vi "Measurement.SetConfiguration.vi"(8 "error in (no error)":errorcluster, 10 "Configuration":variant, 11 "Measurement.WavelengthSweeping in":refnum<class "Measurement.WavelengthSweeping.lvclass">) -> (0 "error out":errorcluster, 3 "Measurement.WavelengthSweeping out":refnum<class "Measurement.WavelengthSweeping.lvclass">)   [LabVIEW 2017, in "Measurement.WavelengthSweeping.lvclass"]
uses:
  Measurement.WavelengthSweeping.lvclass
  Typedefs/Configuration--Cluster.ctl
  Measurement/Typedefs/Measurement.Type--Enum.ctl
  Typedefs/Configuration.Hardware--Cluster.ctl
  Measurement/Typedefs/Configuration.SMU--Cluster.ctl
  SMU/Typedefs/Configuration--Cluster.ctl
  Measurement/Typedefs/Configuration.LIA--Cluster.ctl
  LIA/Typedefs/Configuration--Cluster.ctl
  Measurement/Typedefs/Configuration.OPM--Cluster.ctl
  OPM/Typedefs/Configuration--Cluster.ctl
  Measurement/Typedefs/Configuration.OPA--Cluster.ctl
  OPA/Typedefs/Configuration--Cluster.ctl
  Typedefs/Configuration.Measurement--Cluster.ctl
  Measurement/Measurement.lvclass
  SMU/SMU.lvclass
  LIA/LIA.lvclass
  OPM/OPM.lvclass
  OPA/OPA.lvclass
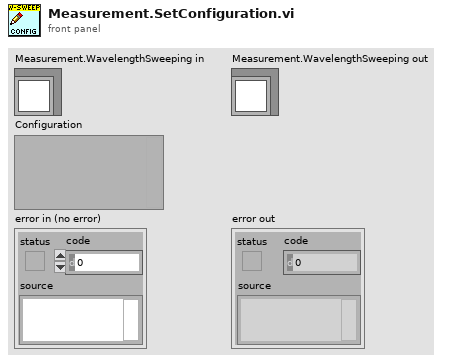
[diagram p1: front panel]
types:
  T1 = typedef "Measurement.WavelengthSweeping.lvclass/Configuration--Cluster.ctl" = cluster{"Measurement.Type":T2, "Hardware":T3, "Measurement":T12}
  T2 = typedef "Measurement.lvclass/Measurement.Type--Enum.ctl" = enum16{"Free", "I/V Curve", "Wavelength sweeping", "Photocurrent mapping"}
  T3 = typedef "Measurement.WavelengthSweeping.lvclass/Configuration.Hardware--Cluster.ctl" = cluster{"SMU":T4, "LIA":T6, "OPM":T8, "OPA":T10}
  T4 = typedef "Measurement.lvclass/Configuration.SMU--Cluster.ctl" = cluster{"Enable":bool, "SMU Model":string, "Configuration":T5}
  T5 = typedef "SMU.lvclass/Configuration--Cluster.ctl" = cluster{"VISA Resource":string, "Channel":string}
  T6 = typedef "Measurement.lvclass/Configuration.LIA--Cluster.ctl" = cluster{"Enable":bool, "LIA Model":string, "Configuration":T7}
  T7 = typedef "LIA.lvclass/Configuration--Cluster.ctl" = cluster{"VISA Resource":string}
  T8 = typedef "Measurement.lvclass/Configuration.OPM--Cluster.ctl" = cluster{"Enable":bool, "OPM Model":string, "Configuration":T9}
  T9 = typedef "OPM.lvclass/Configuration--Cluster.ctl" = cluster{"VISA Resource":string}
  T10 = typedef "Measurement.lvclass/Configuration.OPA--Cluster.ctl" = cluster{"Enable":bool, "OPA Model":string, "Configuration":T11}
  T11 = typedef "OPA.lvclass/Configuration--Cluster.ctl" = cluster{"Serial Number":string}
  T12 = typedef "Measurement.WavelengthSweeping.lvclass/Configuration.Measurement--Cluster.ctl" = cluster{"SMU Voltage, V":dbl, "OPA Start wavelength, nm":dbl, "OPA Stop wavelength, nm":dbl, "OPA Scan resolution, nm":dbl, "OPA Number or points":u16, "Integration time, sec":dbl, "Delay time, ms":u16, "Accumulation":u16}
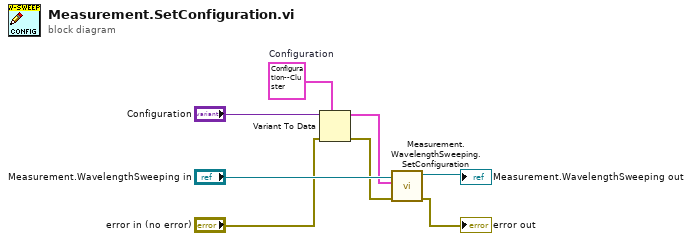
[diagram p0: block diagram]
diagram:
  w7 = T1 {"Measurement.Type"=enum."Free", "Hardware"={"SMU"={"Enable"=FALSE, "SMU Model"="", "Configuration"={"VISA Resource"="", "Channel"=""}}, "LIA"={"Enable"=FALSE, "LIA Model"="", "Configuration"={"VISA Resource"=""}}, "OPM"={"Enable"=FALSE, "OPM Model"="", "Configuration"={"VISA Resource"=""}}, "OPA"={"Enable"=FALSE, "OPA Model"="", "Configuration"={"Serial Number"=""}}}, "Measurement"={"SMU Voltage, V"=0.0, "OPA Start wavelength, nm"=0.0, "OPA Stop wavelength, nm"=0.0, "OPA Scan resolution, nm"=0.0, "OPA Number or points"=0, "Integration time, sec"=0.0, "Delay time, ms"=0, "Accumulation"=0}}  # Configuration
  n1 = Variant To Data(error in="error in (no error)", type=w7, Variant="Configuration") -> (data=w4:T1, error out=w3:errorcluster)
  n2 = call "Measurement.WavelengthSweeping.SetConfiguration.vi"("error in (no error)"=w3, "Configuration"=w4, "Measurement.WavelengthSweeping"="Measurement.WavelengthSweeping in") -> ("error out"=→"error out":errorcluster, "Measurement.WavelengthSweeping out"=→"Measurement.WavelengthSweeping out":refnum<class "Measurement.WavelengthSweeping.lvclass">)  [unwired: 7 in]
